vi "lvUpdateProjectFiles.vi"() -> ()   [LabVIEW 2015, in "veristand-steps-codegen.lvlib"]
uses:
  veristand-steps-codegen.lvlib
  <vilib>/Wiresmith Technology/LabVIEW CLI/CLI Class/CLI.lvclass
panel:
  out "error out":errorcluster
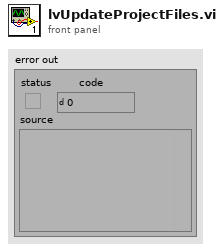
[diagram p1: front panel]
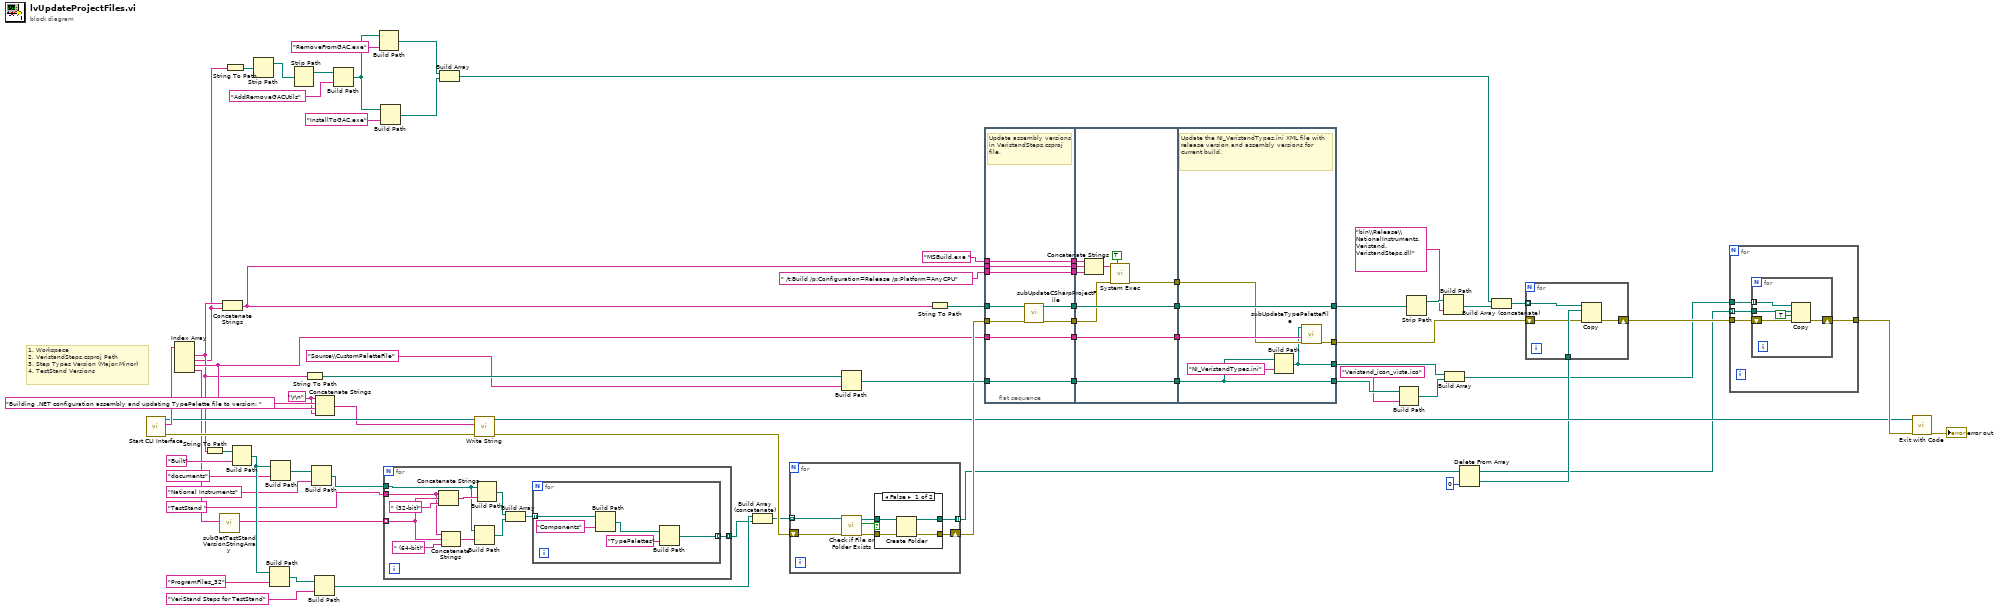
[diagram p0: block diagram]
diagram:
  w44 = "\r\n"
  # "1. Workspace\n2. VeristandSteps.csproj Path\n3. Step Types Version (Major.Minor)\n4. TestStand Versions"
  n1 = call <vilib>:"Start CLI Interface.vi"() -> ("error out"=w51:errorcluster, "Custom Parameters"=w73:string[], "CLI out"=w50:refnum<class "CLI.lvclass">)  [unwired: 9 in]
  n2 = Index Array(array=w73) -> (element #1=w40:string, element #2=w13:string, element #3=w47:string, element #4=w35:string)  [unwired: 4 in]
  n3 = String To Path(string=w40) -> (path=w71:path)
  n4 = call "subGetTestStandVersionStringArray.vi"("TestStand Version String"=w35) -> ("TestStand Version String Array"=w34:string[])  [unwired: 10 in]
  n5 = Concatenate Strings(w40, w13) -> (w64:string)
  n6 = String To Path(string=w13) -> (path=w12:path)
  n7 = Build Path(base path=w71, name or relative path="Built") -> (appended path=w39:path)
  n8 = Strip Path(path=w12) -> (stripped path=w11:path)  [unwired: 1 out]
  n9 = Build Path(base path=w39, name or relative path="ProgramFiles_32") -> (appended path=w32:path)
  n10 = Build Path(base path=w39, name or relative path="documents") -> (appended path=w37:path)
  n11 = Strip Path(path=w11) -> (stripped path=w10:path)  [unwired: 1 out]
  n12 = String To Path(string=w40) -> (path=w67:path)
  n13 = Build Path(base path=w37, name or relative path="National Instruments") -> (appended path=w23:path)
  n14 = Build Path(base path=w32, name or relative path="VeriStand Steps for TestStand") -> (appended path=w21:path)
  n15 = Concatenate Strings(w44, "Building .NET configuration assembly and updating TypePalette file to version: " ("string"), w47, w44) -> (w46:string)
  n16 = Build Path(base path=w10, name or relative path="AddRemoveGACUtils") -> (appended path=w7:path)
  n17 = Build Path(base path=w7, name or relative path="RemoveFromGAC.exe") -> (appended path=w4:path)
  n18 = Build Path(base path=w7, name or relative path="InstallToGAC.exe") -> (appended path=w3:path)
  n19 = for {
    tunnel: w34 -> [w83] mode=indexing
    tunnel: w23 -> [w80]
    tunnel: "TestStand " ("name or relative path") -> [w79]
    tunnel: [w75] -> w14 mode=concatenating
    n20 = Concatenate Strings(w79, w83, " (32-bit)" ("string")) -> (w81:string)
    n21 = Concatenate Strings(w79, w83, " (64-bit)" ("string")) -> (w82:string)
    n22 = Build Path(base path=w80, name or relative path=w82) -> (appended path=w77:path)
    n23 = Build Path(base path=w80, name or relative path=w81) -> (appended path=w78:path)
    n24 = Build Array(w78, w77) -> (w76:path[])
    n25 = for {
      tunnel: w76 -> [w90] mode=indexing
      tunnel: [w86] -> w75 mode=indexing
      n26 = Build Path(base path=w90, name or relative path="Components") -> (appended path=w88:path)
      n27 = Build Path(base path=w88, name or relative path="TypePalettes") -> (appended path=w86:path)
    }
  }
  n28 = Build Array(w4, w3) -> (w2:path[])
  n29 = call <vilib>:"Write String.vi"("error in (no error)"=w51, "Text to Write"=w46, "CLI in"=w50) -> ("error out"=w49:errorcluster, "CLI out"=w48:refnum<class "CLI.lvclass">)  [unwired: 7 in]
  n30 = Build Array (concatenate)(w21, w14) -> (w30:path[])
  n31 = for {
    tunnel: [w93] -> w28 mode=indexing
    shift-right: [w94] -> w54
    shift-left: w49 -> [w92]
    tunnel: w30 -> [w91] mode=indexing
    n32 = call <vilib>:"Check if File or Folder Exists.vi"("error in (no error)"=w92, "path"=w91) -> ("error out"=w97:errorcluster, "file or folder exists?"=w95:bool, "dup path"=w96:path)  [unwired: 7 in]
    n33 = case shown="False" w95 {
      tunnel: w97 -> [w101 w102]
      tunnel: w96 -> [w100 w103]
      tunnel: [w99 w102] -> w94
      tunnel: [w98 w103] -> w93
      frame False {
        n34 = Create Folder(path (use dialog)=w100, error in=w101) -> (created path=w98:path, error out=w99:errorcluster)  [unwired: 1 in, 1 out]
      }
      frame True {
      }
    }
  }
  n35 = Build Path(base path=w67, name or relative path="Source\\CustomPaletteFile") -> (appended path=w56:path)
  n36 = String To Path(string=w64) -> (path=w60:path)
  n37 = flat-sequence {
    tunnel: w64 -> [w110]
    tunnel: " /t:Build /p:Configuration=Release /p:Platform=AnyCPU" ("string") -> [w111]
    tunnel: "MSBuild.exe " -> [w112]
    tunnel: [w112] -> w63
    tunnel: [w111] -> w62
    tunnel: [w110] -> w61
    tunnel: w60 -> [w109]
    tunnel: [w108] -> w59
    tunnel: [w107] -> w58
    tunnel: w56 -> [w106]
    tunnel: [w106] -> w55
    tunnel: w54 -> [w105]
    tunnel: w47 -> [w104]
    tunnel: [w104] -> w53
    tunnel: [w122] -> w43
    tunnel: [w121] -> w42
    tunnel: [w120] -> w41
    tunnel: w53 -> [w120]
    tunnel: w55 -> [w121]
    tunnel: w58 -> [w122]
    tunnel: w59 -> [w114]
    tunnel: w61 -> [w116]
    tunnel: w62 -> [w117]
    tunnel: w63 -> [w118]
    tunnel: [w113] -> w29
    tunnel: [w129] -> w57
    tunnel: w43 -> [w129]
    tunnel: w42 -> [w126]
    tunnel: [w128] -> w16
    tunnel: [w126] -> w20
    tunnel: w41 -> [w125]
    tunnel: w29 -> [w124]
    tunnel: [w123] -> w18
    frame #0 {
      # "Update assembly versions in VeristandSteps.csproj file."
      n38 = call "subUpdateCSharpProjectFile.vi"("error in (no error)"=w105, ".csproj path"=w109) -> ("error out"=w108:errorcluster, ".csproj path out"=w107:path)  [unwired: 8 in]
    }
    frame #1 {
      n39 = Concatenate Strings(w118, w116, w117) -> (w115:string)
      n40 = call <vilib>:"System Exec.vi"("wait until completion? (T)"=TRUE, "error in (no error)"=w114, "command line"=w115) -> ("error out"=w113:errorcluster)  [unwired: 5 in, 3 out]
    }
    frame #2 {
      # "Update the NI_VeristandTypes.ini XML file with release version and assembly versions for current build."
      n41 = Build Path(base path=w126, name or relative path="NI_VeristandTypes.ini") -> (appended path=w123:path)
      n42 = call "subUpdateTypePaletteFile.vi"("error in (no error)"=w124, "Step Types Version"=w125, "TypePalette .ini file location"=w123) -> ("error out"=w128:errorcluster)  [unwired: 8 in]
    }
  }
  n43 = Build Path(base path=w20, name or relative path="Veristand_icon_vista.ico") -> (appended path=w17:path)
  n44 = Strip Path(path=w57) -> (stripped path=w69:path)  [unwired: 1 out]
  n45 = Build Path(base path=w69, name or relative path="bin\\Release\\NationalInstruments.Veristand.VeristandSteps.dll") -> (appended path=w8:path)
  n46 = Build Array(w18, w17) -> (w15:path[])
  n47 = Delete From Array(array=w28, index=0) -> (deleted portion=w26:path, array with subset deleted=w25:path[])  [unwired: 1 in]
  n48 = Build Array (concatenate)(w2, w8) -> (w1:path[])
  n49 = for {
    tunnel: w26 -> [w132]
    shift-right: [w133] -> w27
    shift-left: w16 -> [w131]
    tunnel: w1 -> [w130] mode=indexing
    n50 = Copy(8:w131, 10:w132, 11:w130) -> (0:w133:errorcluster)  [unwired: 2 in, 2 out]
  }
  n51 = for {
    tunnel: [w137] -> w65
    tunnel: w27 -> [w136]
    tunnel: w25 -> [w135] mode=indexing
    tunnel: w15 -> [w134]
    n52 = for {
      tunnel: w135 -> [w140]
      shift-right: [w142] -> w137
      shift-left: w136 -> [w141]
      tunnel: w134 -> [w138] mode=indexing
      n53 = Copy(8:w141, 9:TRUE ("overwrite (F)"), 10:w140, 11:w138) -> (0:w142:errorcluster)  [unwired: 1 in, 2 out]
    }
  }
  n54 = call <vilib>:"Exit with Code.vi"("error in (no error)"=w65, "CLI in"=w48) -> ("error out"=→"error out":errorcluster)  [unwired: 9 in]
